vi "Get Class.vi"(8 "error in (no error)":errorcluster, 11 "DSFPlugin Transceiver in":refnum<class "DSFPlugin Transceiver.lvclass">) -> (0 "error out":errorcluster, 2 "class":string, 3 "DSFPlugin Transceiver out":refnum<class "DSFPlugin Transceiver.lvclass">)   [LabVIEW 2017, in "DSFPluginTest.lvlib" / "DSFPlugin Transceiver.lvclass"]
uses:
  DSFPlugin Transceiver.lvclass
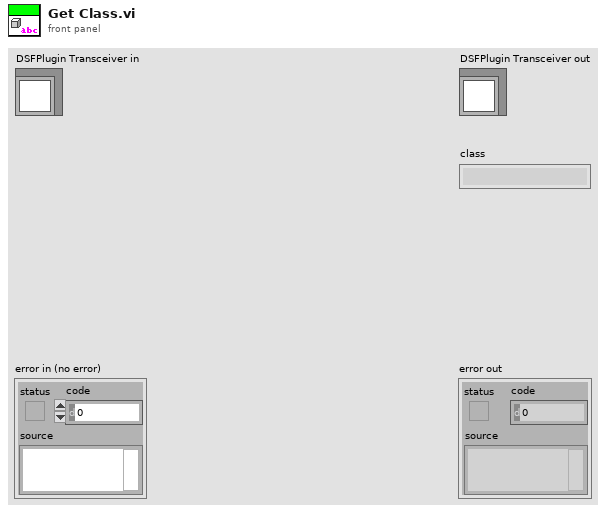
[diagram p1: front panel]
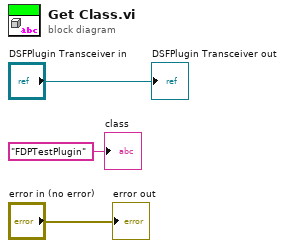
[diagram p0: block diagram]
diagram:
  "error out" <- "error in (no error)"
  "DSFPlugin Transceiver out" <- "DSFPlugin Transceiver in"
  "class" <- "FDPTestPlugin" ("class")
